vi "getOutputState.vi"(7 "chn":string, 8 "error in (no error)":errorcluster, 11 "PsuNiPxi in":refnum<class "PsuNi.lvclass">) -> (0 "error out":errorcluster, 2 "state":bool, 3 "PsuNiPxi out":refnum<class "PsuNi.lvclass">)   [LabVIEW 2023, in "PsuNi.lvclass"]
doc: "<b>Author:</b> Wolfgang\n<b>Description:</b> get output state of power supply by channel, true = on; false = off"
uses:
  PsuNi.lvclass
  PsuNi.lvclass/PsuNi.ctl
  <instrlib>/niDCPower/nidcpower.llb/niDCPower Output State.ctl
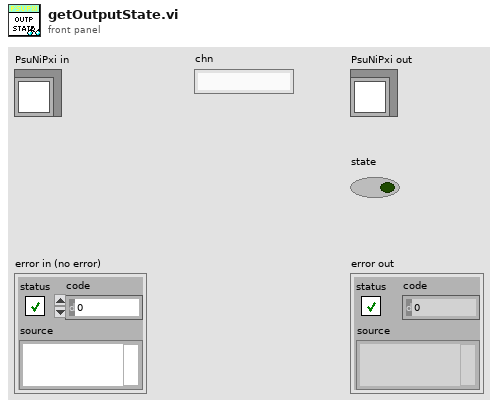
[diagram p1: front panel]
types:
  T1 = typedef "niDCPower Output State.ctl" = u16
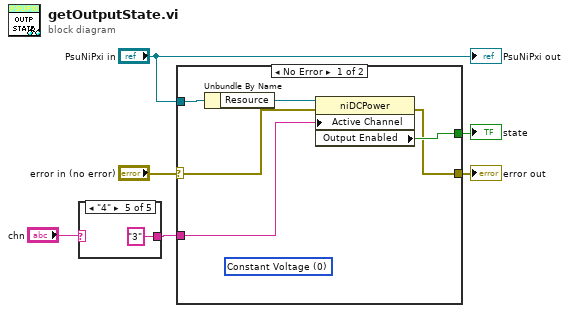
[diagram p0: block diagram]
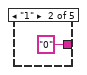
[diagram p3: hidden frame]
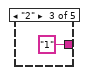
[diagram p4: hidden frame]
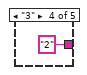
[diagram p5: hidden frame]
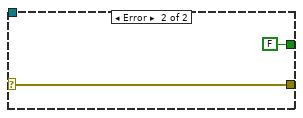
[diagram p6: hidden frame]
diagram:
  n1 = case shown="\"4\"" "chn" {
    selector: "chn" -> [w7 _ _ _ _]
    tunnel: [w7 "0" "1" "2" "3"] -> w2
    frame "False", Default {
    }
    frame "1" {
    }
    frame "2" {
    }
    frame "3" {
    }
    frame "4" {
    }
  }
  n2 = case shown="No Error" "error in (no error)" {
    selector: "error in (no error)" -> [w12 w19]
    tunnel: [w14 FALSE ("in state?")] -> w6
    tunnel: w2 -> [w15 _]
    tunnel: [w13 w19] -> w4
    tunnel: "PsuNiPxi in" -> [w17 _]
    frame No Error {
      (unwired) T1 0 items=["Constant Voltage", "Constant Current"] ("output state")
      n3 = Unbundle By Name(w17) -> ("Resource"=w16:refnum<k15>)
      n4 = property class="niDCPower"(reference=w16, error in=w12, "Active Channel"=w15) -> (error out=w13:errorcluster, "Output Enabled"=w14:bool)  [unwired: 1 out]
    }
    frame Error {
    }
  }
  "error out" <- w4
  "state" <- w6
  "PsuNiPxi out" <- "PsuNiPxi in"
